vi "Execution Loop.vi"(11 "Array":string[](array[string])) -> (0 "error out":errorcluster, 3 "resul":i64)   [LabVIEW 2020]
uses:
  <vilib>/ErrorRing/Error Ring.xnode
  <vilib>/Utility/error.llb/Error Cluster From Error Code.vi
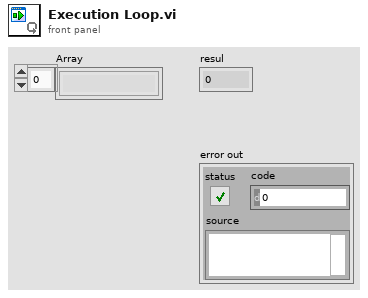
[diagram p1: front panel]
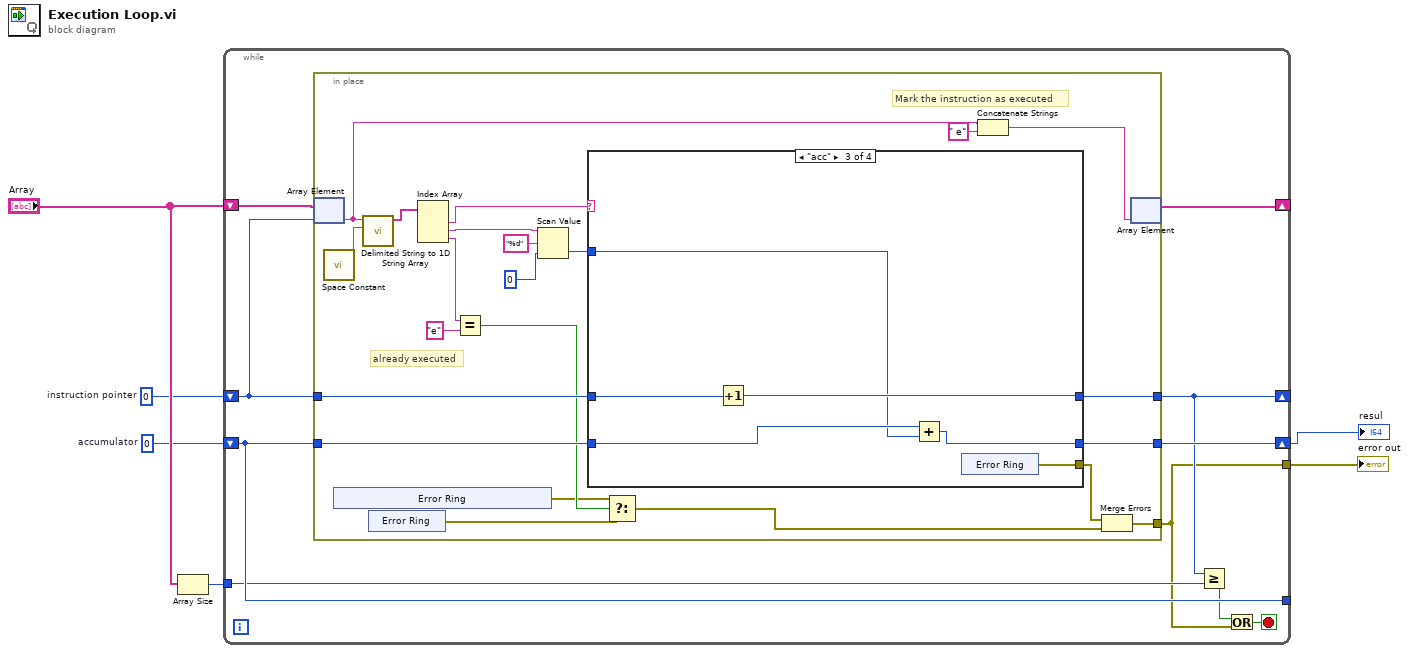
[diagram p0: block diagram]
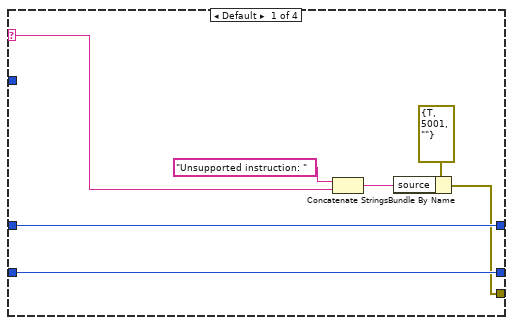
[diagram p2: hidden frame]
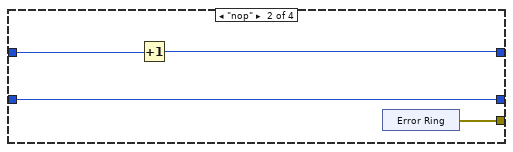
[diagram p3: hidden frame]
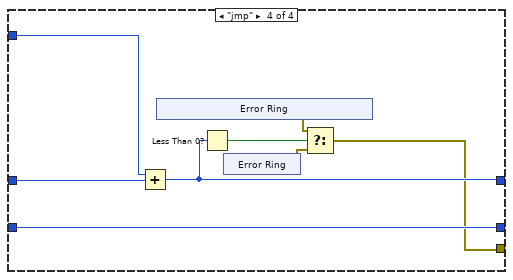
[diagram p4: hidden frame]
diagram:
  w2 = i64 0  # instruction pointer
  w1 = i64 0  # accumulator
  n1 = Array Size(array="Array") -> (size(s)=w5:i32)
  n2 = while {
    shift-right: [w15] -> w6
    shift-left: w1 -> [w16]
    tunnel: [w16] -> _
    shift-right: [w11] -> _
    shift-left: w2 -> [w13]
    shift-right: [w12] -> _
    shift-left: "Array" -> [w14]
    tunnel: [w7] -> w3
    tunnel: w5 -> [w10]
    stop <- w9 stop-if-true
    n3 = in-place {
      in-place-border: w16 -> [w38]
      in-place-border: [w37] -> w15
      in-place-border: [w36] -> w11
      in-place-border: w13 -> [w35]
      in-place-border: [w27] -> w7
      # "Mark the instruction as executed"
      # "already executed"
      n4 = in-place-array #1(w14, w13) -> (w25:string)
      n5 = call <vilib>:"Space Constant.vi"() -> ("String"=w31:string)
      n6 = xnode "Error Ring"() -> ("error out"=w18:errorcluster)
      n7 = call <vilib>:"Delimited String to 1D String Array.vi"("delimiter"=w31, "delimited string"=w25) -> ("string array"=w30:string[])  [unwired: 9 in]
      n8 = xnode "Error Ring"() -> ("error out"=w19:errorcluster)
      n9 = Index Array(array=w30) -> (element #1=w29:string, element #2=w28:string, element #3=w22:string)  [unwired: 3 in]
      n10 = Equal?(x=w22, y="e") -> (x = y?=w20:bool)
      n11 = Scan Value(string=w28, format string="%d", default (0 dbl)=i64 0) -> (value=w33:i64)  [unwired: 1 out]
      n12 = case shown="\"acc\"" w29 {
        selector: w29 -> [w46 _ _ _]
        tunnel: w38 -> [w51 w55 w62 w71]
        tunnel: [w51 w55 w58 w71] -> w37
        tunnel: w35 -> [w50 w54 w61 w70]
        tunnel: [w50 w53 w60 w68] -> w36
        tunnel: w33 -> [_ _ w57 w69]
        tunnel: [w45 w52 w59 w64] -> w26
        frame Default {
          n13 = Concatenate Strings("Unsupported instruction: " ("source 2"), w46) -> (w48:string)
          n14 = Bundle By Name(cluster=errorcluster {"status"=TRUE, "code"=5001, "source"=""} ("error constant"), "source"=w48) -> (w45:errorcluster)
        }
        frame "nop" {
          n15 = Increment(x=w54) -> (x+1=w53:i64)
          n16 = xnode "Error Ring"() -> ("error out"=w52:errorcluster)
        }
        frame "acc" {
          n17 = Increment(x=w61) -> (x+1=w60:i64)
          n18 = Add(x=w62, y=w57) -> (x+y=w58:i64)
          n19 = xnode "Error Ring"() -> ("error out"=w59:errorcluster)
        }
        frame "jmp" {
          n20 = Add(x=w69, y=w70) -> (x+y=w68:i64)
          n21 = xnode "Error Ring"() -> ("error out"=w65:errorcluster)
          n22 = Less Than 0?(x=w68) -> (x < 0?=w67:bool)
          n23 = xnode "Error Ring"() -> ("error out"=w66:errorcluster)
          n24 = Select(t=w65, s=w67, f=w66) -> (s? t:f=w64:errorcluster)
        }
      }
      n25 = Select(t=w18, s=w20, f=w19) -> (s? t:f=w17:errorcluster)
      n26 = Concatenate Strings(w25, " e" ("string")) -> (w23:string)
      n27 = Merge Errors(w26, w17) -> (w27:errorcluster)
      n28 = in-place-array #1(w23) -> (w12:string[])  [unwired: 1 out]
    }
    n29 = Greater Or Equal?(x=w11, y=w10) -> (x >= y?=w8:bool)
    n30 = Or(x=w8, y=w7) -> (x .or. y?=w9:bool)
  }
  "resul" <- w6
  "error out" <- w3
